vi "Function File List.vi"(8 "error in (no error)":errorcluster, 11 "Function Type":T1) -> (0 "error out":errorcluster, 3 "Function Paths":path[](array[path]))   [LabVIEW 2013]
doc: "Creates an array of function paths based on the function type (Position or Velocity)."
uses:
  Function File List Enum.ctl
  HHMI - Filepaths global.vi
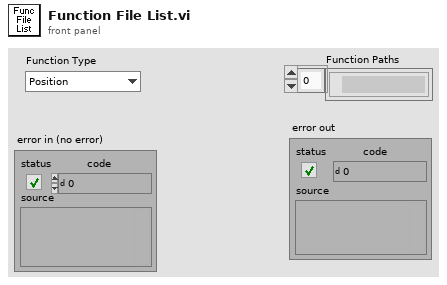
[diagram p1: front panel]
types:
  T1 = typedef "Function File List Enum.ctl" = enum16{"Position", "Velocity"}
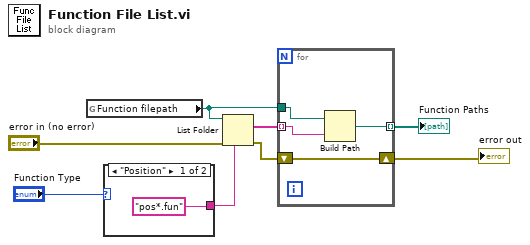
[diagram p0: block diagram]
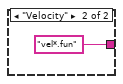
[diagram p2: hidden frame]
diagram:
  n1 = global read "HHMI - Filepaths global.vi" "Function filepath"() -> (w2:path)
  n2 = case shown="\"Position\"" "Function Type" {
    tunnel: ["pos*.fun" ("pattern") "vel*.fun" ("pattern")] -> w1
    frame "Position" {
    }
    frame "Velocity" {
    }
  }
  n3 = List Folder(path=w2, pattern=w1, error in="error in (no error)") -> (filenames=w8:string[], error out=w5:errorcluster)  [unwired: 1 in, 2 out]
  n4 = for {
    tunnel: w8 -> [w13] mode=indexing
    tunnel: w2 -> [w14]
    tunnel: [w12] -> w7 mode=indexing
    shift-right: [w11] -> w4
    shift-left: w5 -> [w11]
    n5 = Build Path(base path=w14, name or relative path=w13) -> (appended path=w12:path)
  }
  "Function Paths" <- w7
  "error out" <- w4
